vi "Live_Plot.vi"() -> ()   [LabVIEW 2013]
uses:
  Private/Controls/Graph.ctl
  Private/Controls/Constraints.ctl
  Private/Controls/Waveforms.ctl
  <vilib>/Utility/miscctls.llb/LVPointTypeDef.ctl
  <userlib>/_OpenG.lib/comparison/comparison.llb/Variant Changed__ogtk.vi
  <userlib>/_OpenG.lib/array/array.llb/Empty 1D Array (Variant)__ogtk.vi
panel:
  out "Cursor grabbed?":bool
  out "Month":dbl
  out "Updating...":bool
  out "Density (g/cc)":dbl=7.874000072479248 min=0.0 max=25.0
  in  "Tab Control":T1(tab)
  out "Number of Matching Events:":i64
  out "Percent of triggers that fit constraints:":dbl format="%#_4g%"
  out "Total Number of triggers:":i64
  in  "Enable\nTimestamp":bool
  out "Constrained Distribution":T2
  in  "Save Image":bool
  in  "Constraints":T3={"Upper Timestamp Range"=timestamp(0 s since 1904-01-01), "Lower Timestamp Range"=timestamp(0 s since 1904-01-01), "Experiment Group:"="", "Experiment Name:"=[], "Upper Velocity Limit (km/s)"=0.0, "Lower Velocity Limit (km/s)"=0.0, "Upper Mass Limit (kg)"=0.0, "Lower Mass Limit (kg)"=0.0, "name array"=[], "Estimate Quality"={0.0, 5.0}} {"Estimate Quality" scale=0.0..5.0; "Lower Mass Limit (kg)" min=0.0 step=1e-20; "Upper Mass Limit (kg)" min=0.0 step=1e-20}
  in  "Velocity":dbl=1.0 min=0.1 max=100.0
  in  "Mass":dbl=2.638602750087072e-13 min=1e-20 max=1e-10
  in  "Radius (µm)":dbl=2.0 min=0.00671912 max=14.4759
  in  "Reset Visible Time":bool caption="Save Metadata"
  in  "Time Visible":dbl=5000.0 min=0.0 max=5000.0 step=100.0
  out "Selected Waveforms":u64[](array[numeric])
  out "Waveforms":T4[](array[typedef])
  out "Max Time":dbl=5000.0
  in  "If this was the big acc...":bool
  out "Max Query Time":dbl
  in  "Pelletron Voltage (MV):":dbl=2.0
  out "Experiment Start":timestamp
  out "Test":bool caption="Test Database in use:"
  out "Test 2":bool caption="Production Database in use:"
  in  "error in (no error)":errorcluster
  out "error out":errorcluster
  in  "Vnoise Estimate:":dbl=0.005
  in  "Sensitivity:":dbl=12100000000000.0
  in  "Update interval (s)":dbl=5.0 min=1.0 max=60.0 step=1.0 format="%#_4g"
  out "Query Time":dbl
  in  "Small?":bool
  in  "Exit":bool
  # "Live Plot of Current Experiment"
  # "Cursor"
  # "Plot Settings:"
  # "ODBC Connection Status:"
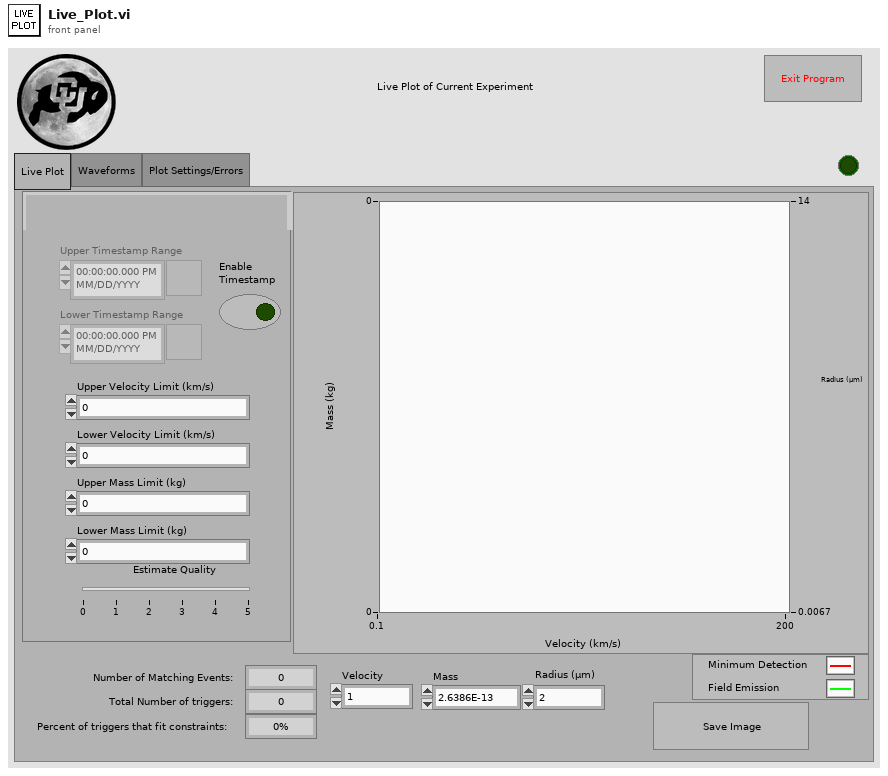
[diagram p1: front panel]
types:
  T1 = enum32{"Live Plot", "Waveforms", "Plot Settings/Errors"}
  T2 = typedef "Graph.ctl" = cluster{cluster{"Vnoise":dbl, "Vnoise":dbl}[]}[]
  T3 = typedef "Constraints.ctl" = cluster{"Upper Timestamp Range":timestamp, "Lower Timestamp Range":timestamp, "Experiment Group:":string, "Experiment Name:":i32[], "Upper Velocity Limit (km/s)":dbl, "Lower Velocity Limit (km/s)":dbl, "Upper Mass Limit (kg)":dbl, "Lower Mass Limit (kg)":dbl, "name array":string[], "Estimate Quality":cluster{dbl, dbl}}
  T4 = typedef "Waveforms.ctl" = cluster{"id_dust_event":u64, "Time Stamp":timestamp, "Velocity":dbl, "Mass":dbl, "Charge":dbl, "Radius":dbl, "Waveform Graph":sgl[][], "Quality":i32}
  T5 = typedef "LVPointTypeDef.ctl" = cluster{"Horizontal":i16, "Vertical":i16}
  T6 = typedef "LVRectTypeDef.ctl" = cluster{"Left":i16, "Top":i16, "Right":i16, "Bottom":i16}
  T7 = enum8{"Enabled", "Disabled", "Disabled and Grayed Out"}
  T8 = typedef "NI_Database_API.lvlib/Conn ObjectReference.ctl" = refnum<k1>
  T9 = typedef "Query_Dust_Event.ctl" = cluster{"Dust Event ID":i64, "Integer Timestamp":i64, "Velocity":sgl, "Mass":sgl, "Charge":sgl, "Radius":sgl, "Passed_3rd_Detector":i8, "High Voltage":sgl, "+ High Voltage Supply":sgl, "- High Voltage Supply":sgl, "HV Control Difference":sgl, "Vacuum Pressure":sgl, "Radiation":sgl, "Column Current":sgl, "Lost Charge":sgl, "Chain Current":sgl, "Control High Voltage":sgl, "Current Group Name:":string, "Current Experiment Name:":string, "Current Experiment Description:":string, "Estimate Source":T10, "Estimate Quality":i8, "File Location":T11, "Dust Type":string, "Dust Density":sgl}
  T10 = typedef "Estimate_source.ctl" = i8
  T11 = typedef "File_location.ctl" = i8
  T12 = typedef "imagedata.ctl" = cluster{"image type":i32, "image depth":i32, "image":u8[], "mask":u8[], "colors":u32[], "Rectangle":cluster{"left":i16, "top":i16, "right":i16, "bottom":i16}}
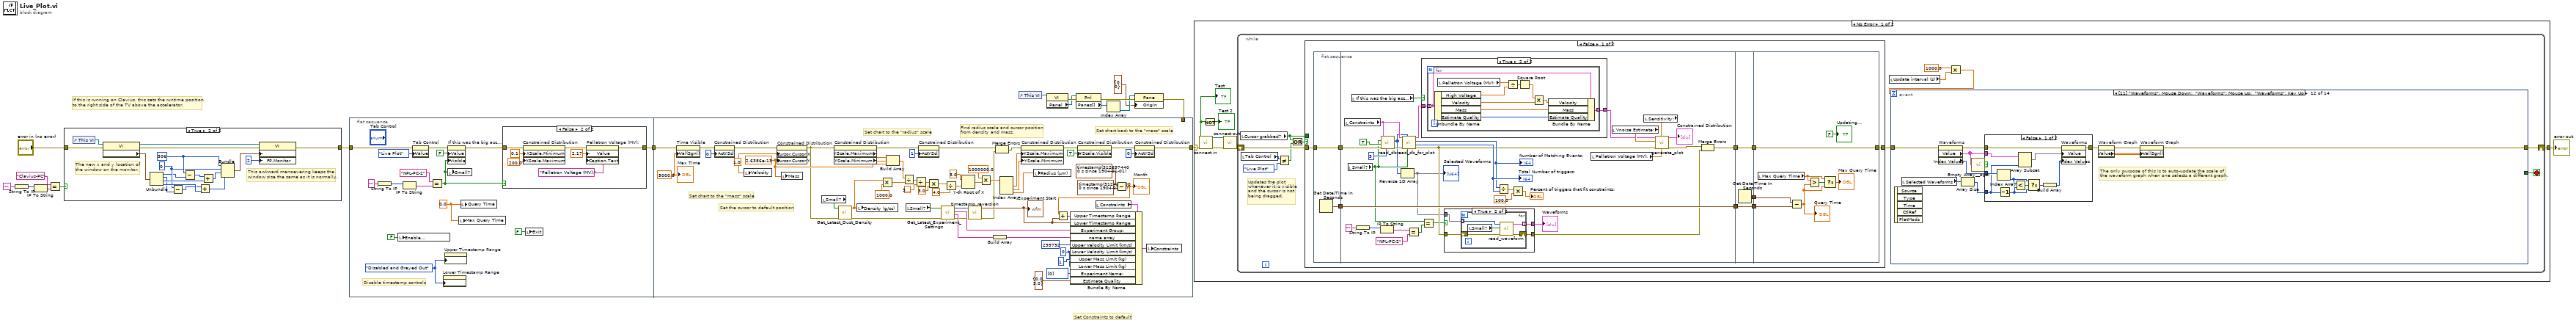
[diagram p0: block diagram]
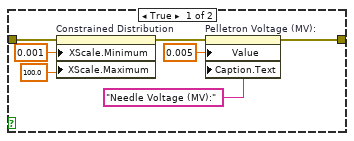
[diagram p3: hidden frame]
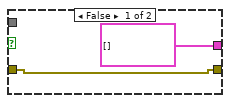
[diagram p4: hidden frame]
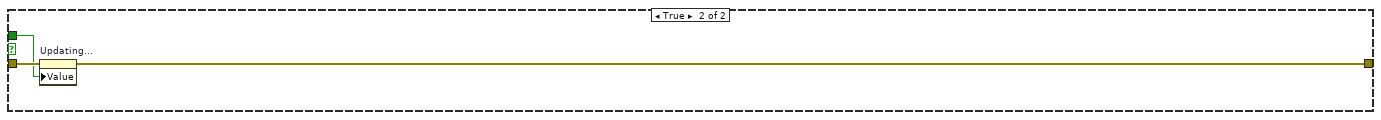
[diagram p6: hidden frame]
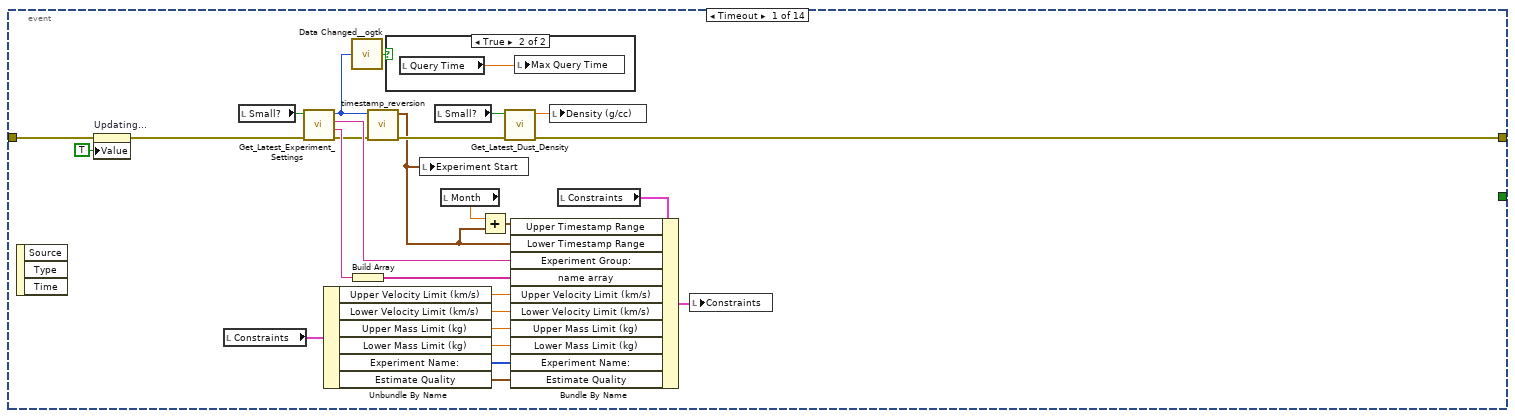
[diagram p7: hidden frame]
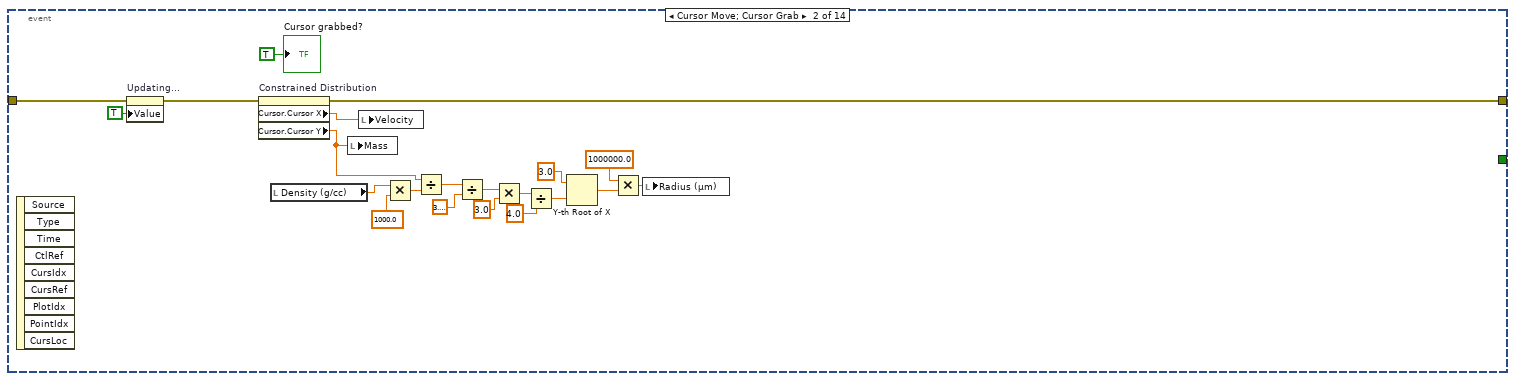
[diagram p9: hidden frame]
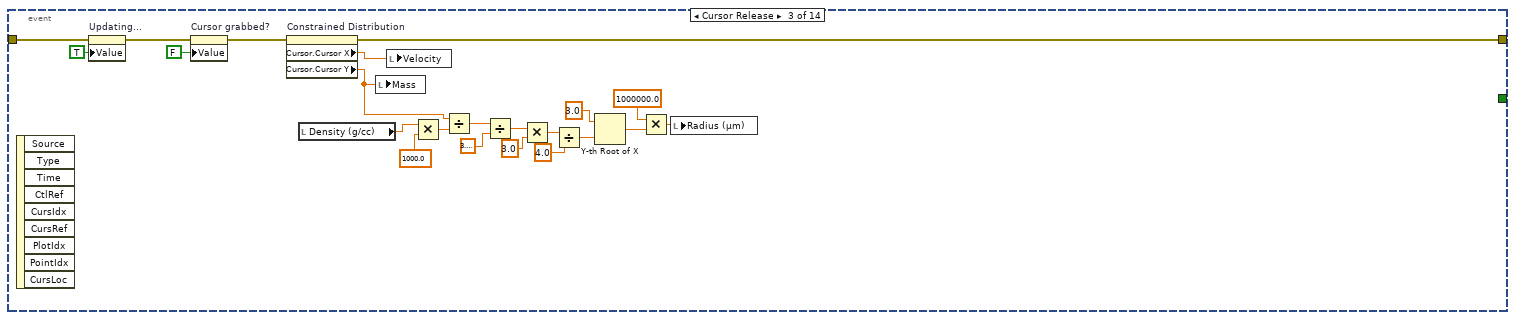
[diagram p10: hidden frame]
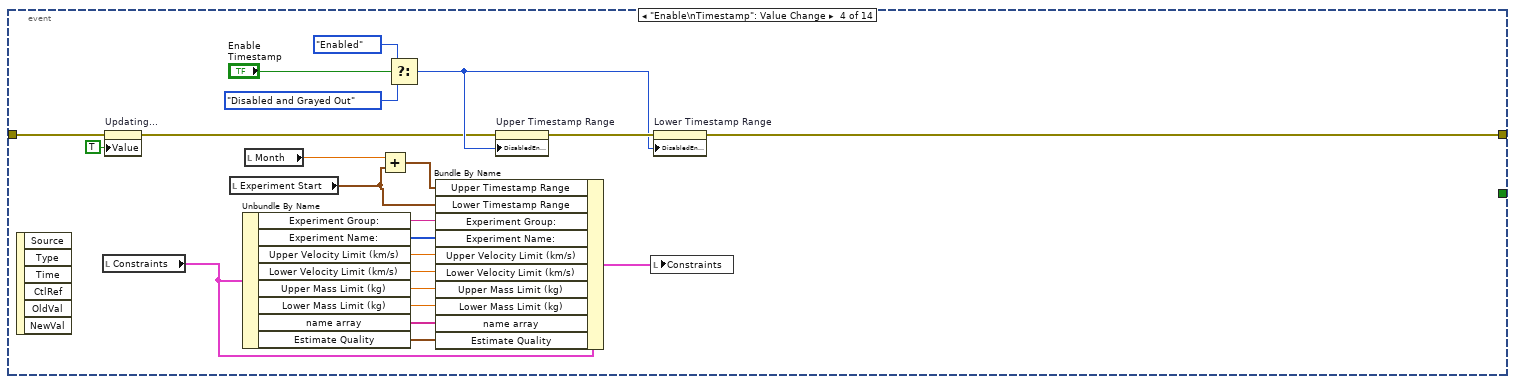
[diagram p11: hidden frame]
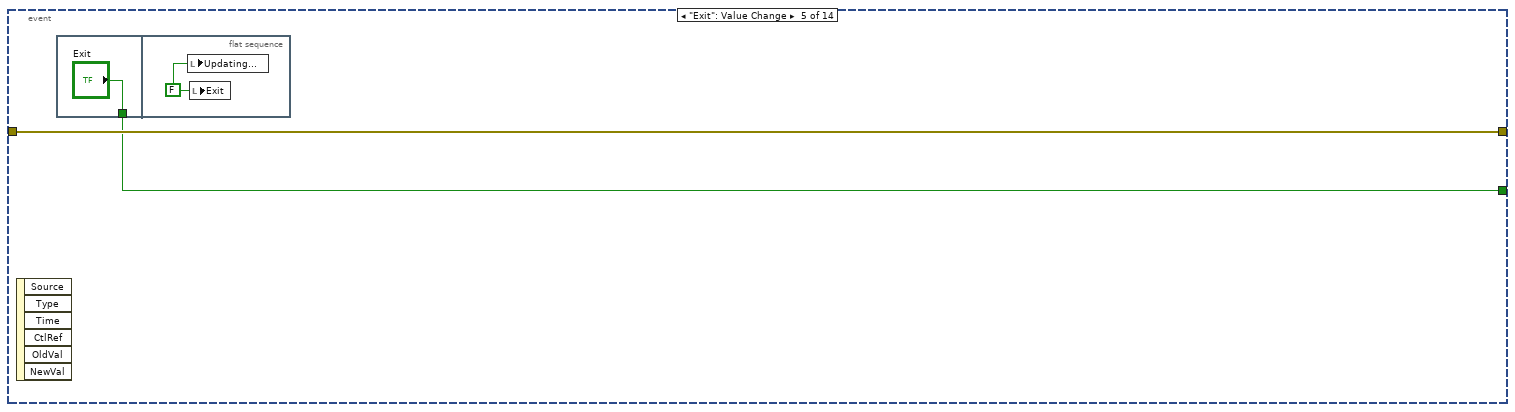
[diagram p12: hidden frame]
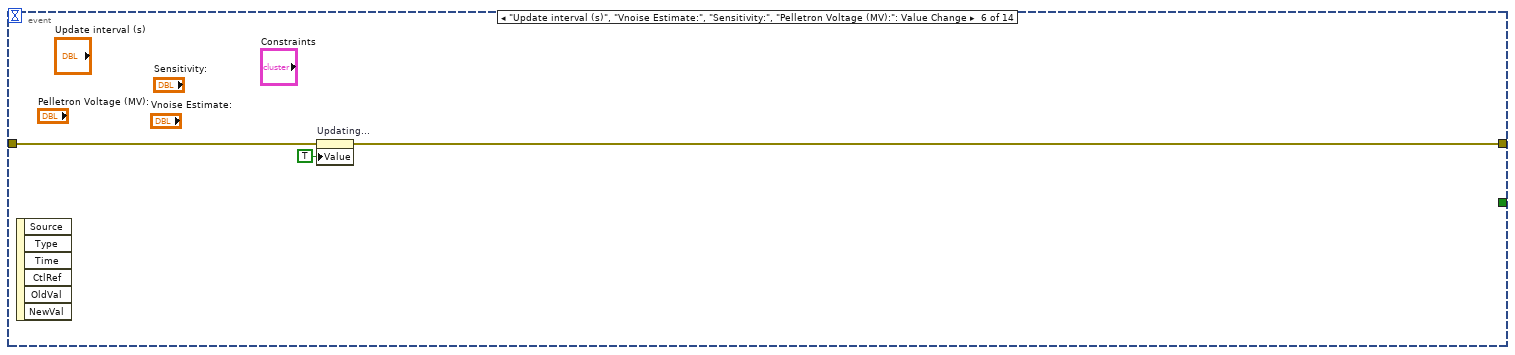
[diagram p13: hidden frame]
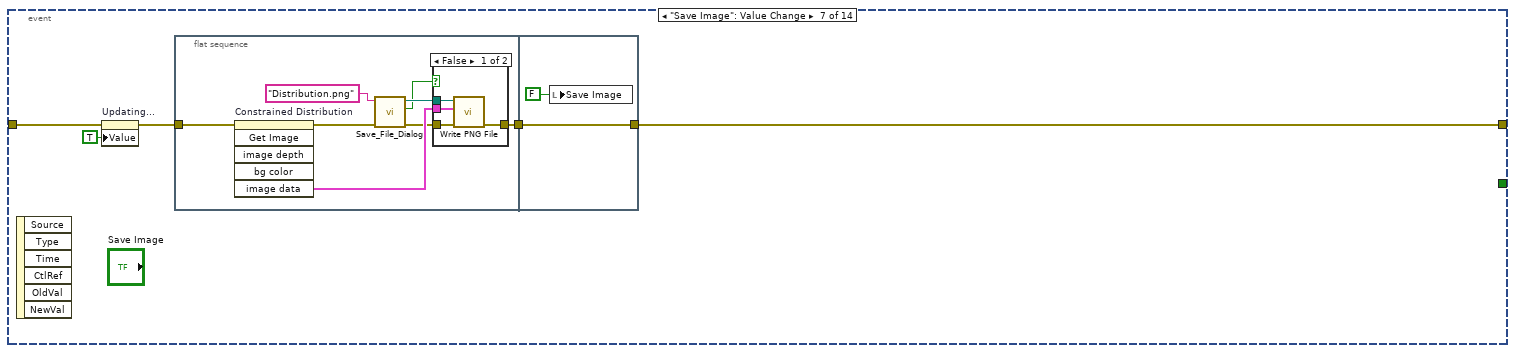
[diagram p14: hidden frame]
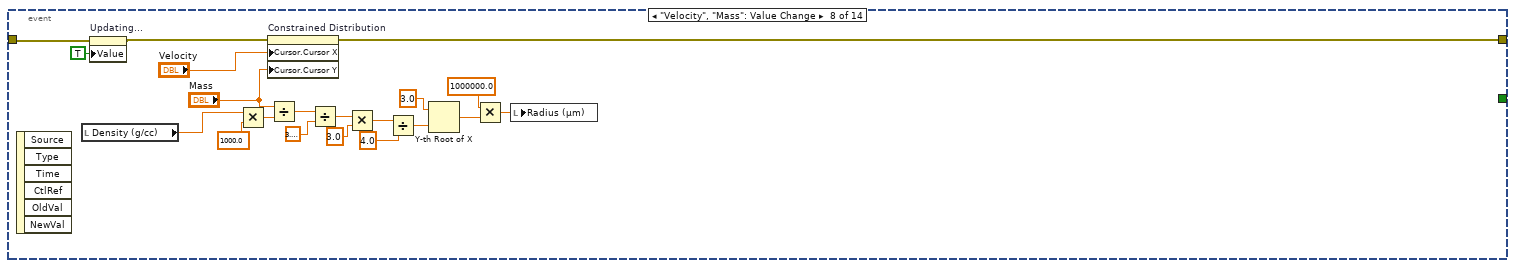
[diagram p16: hidden frame]
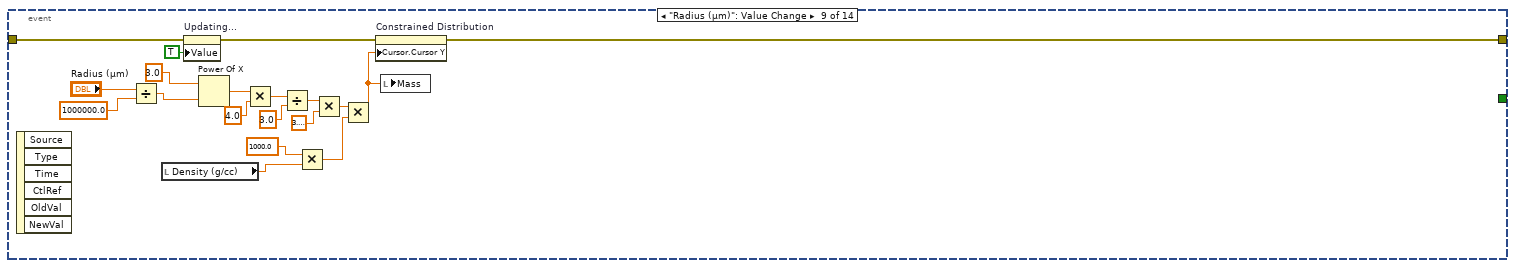
[diagram p17: hidden frame]
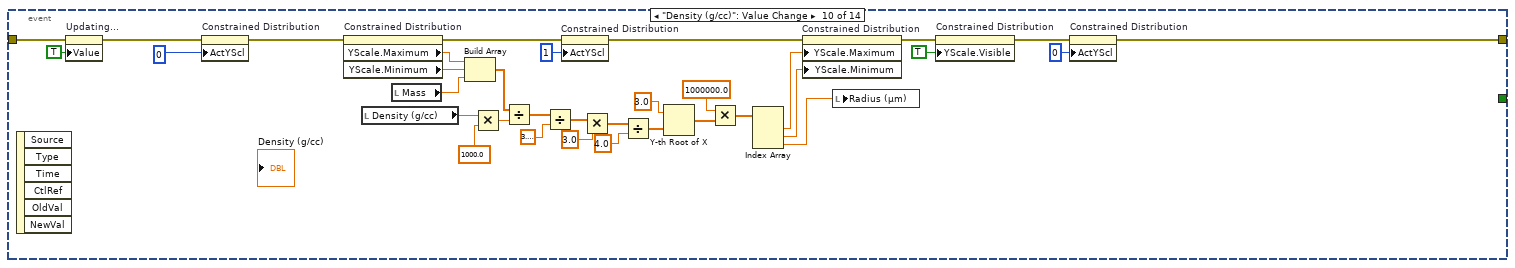
[diagram p18: hidden frame]
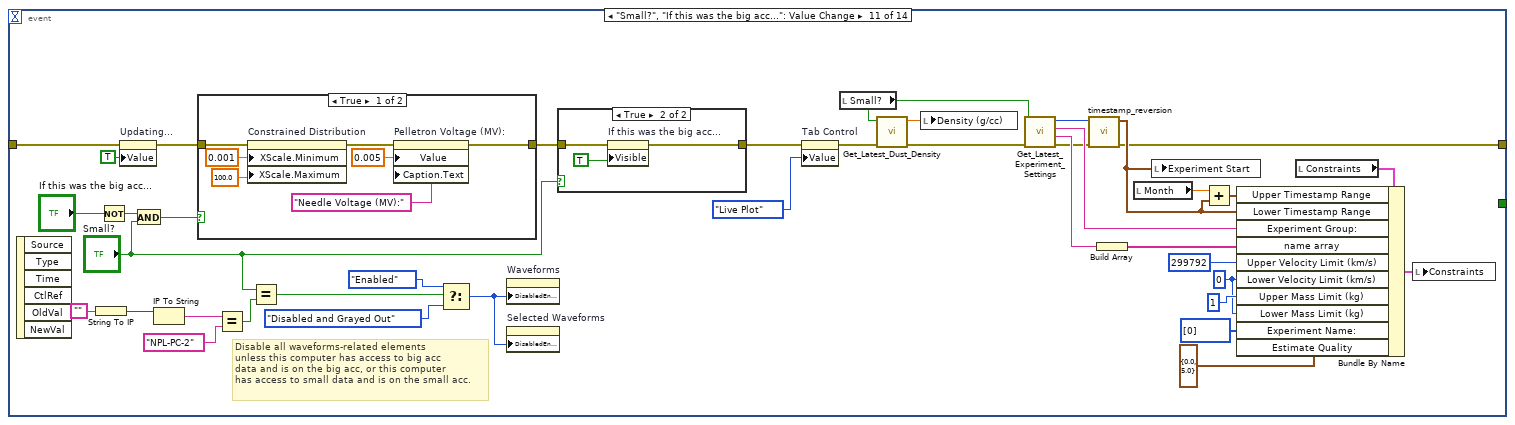
[diagram p19: hidden frame]
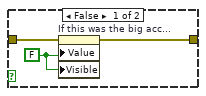
[diagram p20: hidden frame]
diagram:
  # "If this is running on Clavius, this sets the runtime position\nto the right side of the TV above the accelerator."
  # "Set Constraints to default"
  n1 = String To IP(1:"" ("name")) -> (0:w5:u32)
  n2 = IP To String(2:w5) -> (0:w3:string)  [unwired: 1 in]
  n3 = Equal?(x="Clavius-PC", y=w3) -> (x = y?=w7:bool)
  n4 = case shown="True" w7 {
    tunnel: "error in (no error)" -> [w19 w22]
    tunnel: [w19 w20] -> w1
    frame False {
    }
    frame True {
      w27 = i16 0 ("Top")
      w28 = i16 506 ("Left")
      # "This awkward manoevering keeps the\nwindow size the same as it is normally."
      # "The new x and y location of\nthe window on the monitor."
      n5 = control-ref of="This VI"() -> (w36:refnum<vi>)
      n6 = property class="VI"(reference=w36, error in=w22) -> (reference out=w32:refnum<vi>, error out=w21:errorcluster, "Front Panel.WinBounds"=w31:T6)
      n7 = Unbundle(w31) -> ("Left"=w26:i16, "Top"=w25:i16, "Right"=w30:i16, "Bottom"=w29:i16)
      n8 = Subtract(x=w27, y=w25) -> (x-y=w24:i16)
      n9 = Subtract(x=w28, y=w26) -> (x-y=w23:i16)
      n10 = Add(x=w24, y=w29) -> (x+y=w33:i16)
      n11 = Add(x=w23, y=w30) -> (x+y=w34:i16)
      n12 = Bundle("Left"=w28, "Top"=w27, w34, w33) -> (w37:cluster{"Left":i16, "Top":i16, i16, i16})  [unwired: 1 in]
      n13 = property class="VI"(reference=w32, error in=w21, "Front Panel.WinBounds"=w37, "FP.Monitor"=u16 2 ("Front Panel Window:Monitor")) -> (error out=w20:errorcluster)  [unwired: 1 out]
    }
  }
  n14 = flat-sequence {
    tunnel: [w48] -> w8
    tunnel: w1 -> [w40]
    tunnel: [w124] -> w10
    tunnel: w9 -> [_]
    tunnel: w8 -> [w69]
    frame #0 {
      w41 = 0.0 ("Query Time")
      w45 = T7."Disabled and Grayed Out" ("Disabled")
      # "Disable timestamp controls"
      n15 = String To IP(1:"" ("name")) -> (0:w51:u32)
      n16 = local write "Enable\nTimestamp"(FALSE ("Enable\nTimestamp")) -> ()
      n17 = IP To String(2:w51) -> (0:w49:string)  [unwired: 1 in]
      n18 = property on="Tab Control" class="TabCtl (strict)"(error in=w40, "Value"=T1."Live Plot" ("Tab Control")) -> (error out=w39:errorcluster)  [unwired: 1 in, 1 out]
      n19 = Equal?(x="NPL-PC-2", y=w49) -> (x = y?=w42:bool)
      n20 = property on="Lower Timestamp Range" class="AbsTime (strict)"("DisabledEnum"=w45) -> ()  [unwired: 2 in, 2 out]
      n21 = property on="Upper Timestamp Range" class="AbsTime (strict)"("DisabledEnum"=w45) -> ()  [unwired: 2 in, 2 out]
      n22 = property on="If this was the big acc..." class="Bool (strict)"(error in=w39, "Value"=FALSE ("If this was the big acc..."), "Visible"=w42) -> (error out=w44:errorcluster)  [unwired: 1 in, 1 out]
      n23 = local write "Small?"(w42) -> ()
      n24 = local write "Max Query Time"(w41) -> ()
      n25 = local write "Query Time"(w41) -> ()
      n26 = case shown="False" w42 {
        tunnel: [w57 w64] -> w48
        tunnel: w44 -> [w54 w61]
        frame True {
          n27 = property on="Constrained Distribution" class="XYGraph (strict)"(error in=w54, "XScale.Minimum"=0.001 ("X Scale.Range:Minimum"), "XScale.Maximum"=100.0 ("X Scale.Range:Maximum")) -> (error out=w53:errorcluster)  [unwired: 1 in, 1 out]
          n28 = property on="Pelletron Voltage (MV):" class="DigNum (strict)"(error in=w53, "Value"=0.005 ("Pelletron Voltage (MV):"), "Caption.Text"="Needle Voltage (MV):") -> (error out=w57:errorcluster)  [unwired: 1 in, 1 out]
        }
        frame False {
          n29 = property on="Constrained Distribution" class="XYGraph (strict)"(error in=w61, "XScale.Minimum"=0.1 ("X Scale.Range:Minimum"), "XScale.Maximum"=200.0 ("X Scale.Range:Maximum")) -> (error out=w60:errorcluster)  [unwired: 1 in, 1 out]
          n30 = property on="Pelletron Voltage (MV):" class="DigNum (strict)"(error in=w60, "Value"=2.17 ("Pelletron Voltage (MV):"), "Caption.Text"="Pelletron Voltage (MV):") -> (error out=w64:errorcluster)  [unwired: 1 in, 1 out]
        }
      }
      n31 = local write "Exit"(FALSE ("Exit")) -> ()
    }
    frame #1 {
      w67 = 5000.0 ("Max Time")
      w123 = 2.6386e-13 ("Mass")
      w107 = 1.0 ("Velocity")
      w116 = 0
      # "Set chart back to the \"mass\" scale"
      # "Set chart to the \"radius\" scale"
      # "Set chart to the \"mass\" scale"
      # "Find radius scale and cursor position\nfrom density and mass."
      # "Set the cursor to default position"
      n32 = property on="Time Visible" class="DigNum (strict)"(error in=w69, "Val(Sgnl)"=w67) -> (error out=w68:errorcluster)  [unwired: 1 in, 1 out]
      n33 = property on="Constrained Distribution" class="XYGraph (strict)"(error in=w68, "ActYScl"=0 ("Active Y Scale")) -> (error out=w75:errorcluster)  [unwired: 1 in, 1 out]
      n34 = local write "Velocity"(w107) -> ()
      n35 = property on="Constrained Distribution" class="XYGraph (strict)"(error in=w75, "Cursor.Cursor X"=w107, "Cursor.Cursor Y"=w123) -> (error out=w77:errorcluster)  [unwired: 1 in, 1 out]
      n36 = local write "Mass"(w123) -> ()
      n37 = local read "Small?"() -> (w74:bool)
      n38 = property on="Constrained Distribution" class="XYGraph (strict)"(error in=w77) -> (error out=w94:errorcluster, "YScale.Maximum"=w93:dbl, "YScale.Minimum"=w92:dbl)  [unwired: 1 in, 1 out]
      n39 = call "Get_Latest_Dust_Density.vi"("error in (no error)"=w77, "Small?"=w74) -> ("error out"=w79:errorcluster, "Density"=w78:dbl)  [unwired: 8 in]
      n40 = local write "Density (g/cc)"(w78) -> ()
      n41 = Multiply(x=w78, y=1000.0) -> (x*y=w98:dbl)
      n42 = Build Array(w93, w92, w123) -> (w91:dbl[])
      n43 = Divide(x=w91, y=w98) -> (x/y=w106:dbl[])
      n44 = local read "Small?"() -> (w73:bool)
      n45 = Divide(x=w106, y=3.141592653589793) -> (x/y=w104:dbl[])
      n46 = property on="Constrained Distribution" class="XYGraph (strict)"(error in=w94, "ActYScl"=1 ("Active Y Scale")) -> (error out=w90:errorcluster)  [unwired: 1 in, 1 out]
      n47 = Multiply(x=w104, y=3.0) -> (x*y=w102:dbl[])
      n48 = call "Get_Latest_Experiment_Settings.vi"("error in (no error)"=w79, "Small?"=w73) -> ("error out"=w80:errorcluster, "Experiment"=w110:string, "Group"=w109:string, "Integer Timestamp"=w108:i64)  [unwired: 5 in, 1 out]
      n49 = Divide(x=w102, y=4.0) -> (x/y=w100:dbl[])
      n50 = Y-th Root of X(1:w100, 2:3.0 ("y")) -> (0:w96:dbl[])
      n51 = call "timestamp_reversion.vi"("error in (no error)"=w80, "Integer Timestamp"=w108) -> ("error out"=w71:errorcluster, "time stamp"=w111:timestamp)  [unwired: 7 in]
      "Experiment Start" <- w111
      n52 = Multiply(x=1000000.0, y=w96) -> (x*y=w88:dbl[])
      n53 = Build Array(w110) -> (w70:string[])
      n54 = Merge Errors(w90, w71) -> (w72:errorcluster)
      n55 = Index Array(array=w88) -> (element #1=w86:dbl, element #2=w85:dbl, element #3=w84:dbl)  [unwired: 3 in]
      n56 = property on="Constrained Distribution" class="XYGraph (strict)"(error in=w72, "YScale.Maximum"=w86, "YScale.Minimum"=w85) -> (error out=w87:errorcluster)  [unwired: 1 in, 1 out]
      n57 = local write "Radius (µm)"(w84) -> ()
      n58 = property on="Constrained Distribution" class="XYGraph (strict)"(error in=w87, "YScale.Visible"=TRUE ("Y Scale.Visible")) -> (error out=w82:errorcluster)  [unwired: 1 in, 1 out]
      n59 = local read "Constraints"() -> (w122:T3)
      n60 = Subtract(x=timestamp(3126974400 s since 1904-01-01) ("current time"), y=timestamp(3124296000 s since 1904-01-01) ("current time")) -> (x-y=w119:dbl)
      "Month" <- w119
      n61 = Add(x=w119, y=w111) -> (x+y=w120:timestamp)
      n62 = Bundle By Name(cluster=w122, "Upper Timestamp Range"=w120, "Lower Timestamp Range"=w111, "Experiment Group:"=w109, "name array"=w70, "Upper Velocity Limit (km/s)"=299792, "Lower Velocity Limit (km/s)"=w116, "Upper Mass Limit (kg)"=1, "Lower Mass Limit (kg)"=w116, "Experiment Name:"=i32[] [0], "Estimate Quality"=cluster{dbl, dbl} {0.0, 5.0}) -> (w121:T3)
      n63 = property on="Constrained Distribution" class="XYGraph (strict)"(error in=w82, "ActYScl"=0 ("Active Y Scale")) -> (error out=w124:errorcluster)  [unwired: 1 in, 1 out]
      n64 = local write "Constraints"(w121) -> ()
      "Max Time" <- w67
    }
  }
  n65 = control-ref of="This VI"() -> (w17:refnum<vi>)
  n66 = property class="VI"(reference=w17) -> (error out=w16:errorcluster, "Panel"=w15:refnum<vi>)  [unwired: 1 in, 1 out]
  n67 = property class="Pnl"(reference=w15, error in=w16) -> (error out=w14:errorcluster, "Panes[]"=w13:refnum<vi>[])  [unwired: 1 out]
  n68 = Index Array(array=w13) -> (element=w12:refnum<vi>)  [unwired: 1 in]
  n69 = property class="Pane"(reference=w12, error in=w14, "Origin"=T5 {"Horizontal"=0, "Vertical"=0}) -> (error out=w9:errorcluster)  [unwired: 1 out]
  n70 = case shown="No Error" w10 {
    selector: w10 -> [w129 w520]
    tunnel: [w127 w520] -> w18
    frame No Error {
      n71 = call "connect in.vi"("error in (no error)"=w129) -> ("error out"=w130:errorcluster, "Database Connection"=w131:T8, "Test Server"=w128:bool)  [unwired: 6 in]
      "Test" <- w128
      n72 = Not(x=w128) -> (.not. x?=→"Test 2":bool)
      n73 = call "connect out.vi"("error in (no error)"=w130, "connection reference"=w131) -> ("error out"=w126:errorcluster)  [unwired: 9 in]
      n74 = while {
        shift-right: [w140] -> w127
        shift-left: w126 -> [w138]
        stop <- w141 stop-if-true
        # "Updates the plot\nwhenever it is visible\nand the cursor is not\nbeing dragged."
        n75 = local read "Cursor grabbed?"() -> (w132:bool)
        n76 = local read "Tab Control"() -> (w136:T1)
        n77 = Not Equal?(x=w136, y=T1."Live Plot") -> (x != y?=w134:bool)
        n78 = Or(x=w132, y=w134) -> (x .or. y?=w135:bool)
        n79 = case shown="False" w135 {
          tunnel: [w145 w222] -> w139
          tunnel: w138 -> [w144 w224]
          tunnel: w132 -> [_ w223]
          frame False {
            n80 = flat-sequence {
              tunnel: w144 -> [w154]
              tunnel: [w154] -> w152
              tunnel: [w153] -> w151
              tunnel: w152 -> [w173]
              tunnel: [w158] -> w150
              tunnel: [w178] -> w149
              tunnel: w151 -> [w178]
              tunnel: w150 -> [w213]
              tunnel: [w213] -> w148
              tunnel: w149 -> [w212]
              tunnel: [w212] -> w147
              tunnel: [w211] -> w146
              tunnel: [w221] -> w145
              tunnel: w148 -> [w221]
              tunnel: w147 -> [w220]
              tunnel: w146 -> [w215]
              frame #0 {
                n81 = Get Date/Time In Seconds() -> (seconds since 1Jan1904=w153:timestamp)
              }
              frame #1 {
                n82 = local read "Constraints"() -> (w171:T3)
                n83 = local read "Small?"() -> (w162:bool)
                n84 = local read "If this was the big acc..."() -> (w174:bool)
                n85 = String To IP(1:"" ("name")) -> (0:w165:u32)
                n86 = IP To String(2:w165) -> (0:w163:string)  [unwired: 1 in]
                n87 = call "read_db.vi"("No. of Events"=u64 5 ("Limit no. of events"), "error in (no error)"=w173, "Limited?"=TRUE, "Small?"=w162, "Constraints"=w171) -> ("error out"=w172:errorcluster, "Dust Event ID Array"=w156:i64[])  [unwired: 2 in, 3 out]
                n88 = Reverse 1D Array(array=w156) -> (reversed array=w155:i64[])
                "Selected Waveforms" <- w155
                n89 = call "read_db_for_plot.vi"("Small?"=w162, "Selected Dust Events"=w156, "error in (no error)"=w172, "Constraints"=w171) -> ("error out"=w168:errorcluster, "Total Number of triggers"=w179:u64, "Number of Matching Events"=w177:u64, "Dust Array"=w176:T9[])  [unwired: 3 in, 1 out]
                "Total Number of triggers:" <- w179
                "Number of Matching Events:" <- w177
                n90 = Equal?(x=w163, y="NPL-PC-2" ("x")) -> (x = y?=w167:bool)
                n91 = case shown="True" w174 {
                  tunnel: w176 -> [w198 w200]
                  tunnel: [w198 w199] -> w175
                  frame False {
                  }
                  frame True {
                    n92 = for {
                      tunnel: w200 -> [w210] mode=indexing
                      tunnel: [w209] -> w199 mode=indexing
                      n93 = Unbundle By Name(w210) -> ("High Voltage"=w205:sgl, "Velocity"=w204:sgl, "Mass"=w207:sgl, "Estimate Quality"=w208:i8)
                      n94 = local read "Pelletron Voltage (MV):"() -> (w206:dbl)
                      n95 = Divide(x=w206, y=w205) -> (x/y=w202:dbl)
                      n96 = Square Root(x=w202) -> (sqrt(x)=w201:dbl)
                      n97 = Multiply(x=w201, y=w204) -> (x*y=w203:dbl)
                      n98 = Bundle By Name(cluster=w210, "Velocity"=w203, "Mass"=w207, "Estimate Quality"=w208) -> (w209:T9)
                    }
                  }
                }
                n99 = Equal?(x=w162, y=w167) -> (x = y?=w161:bool)
                n100 = case shown="True" w161 {
                  tunnel: w168 -> [w187 w192]
                  tunnel: [T4[] [] ("Waveforms") w191] -> w160
                  tunnel: [w187 w190] -> w157
                  tunnel: w155 -> [_ w189]
                  frame False {
                  }
                  frame True {
                    n101 = for {
                      tunnel: [w195] -> w191 mode=indexing
                      shift-right: [w194] -> w190
                      shift-left: w192 -> [w196]
                      tunnel: w189 -> [w193] mode=indexing
                      n102 = local read "Small?"() -> (w197:bool)
                      n103 = call "read_waveform.vi"("error in (no error)"=w196, "Small?"=w197, "Dust Event ID"=w193) -> ("error out"=w194:errorcluster, "Waveform"=w195:T4)  [unwired: 7 in]
                    }
                  }
                }
                "Waveforms" <- w160
                n104 = Divide(x=w177, y=w179) -> (x/y=w182:dbl)
                n105 = Multiply(x=w182, y=100.0) -> (x*y=→"Percent of triggers that fit constraints:":dbl)
                n106 = local read "Pelletron Voltage (MV):"() -> (w183:dbl)
                n107 = local read "Vnoise Estimate:"() -> (w184:dbl)
                n108 = local read "Sensitivity:"() -> (w185:dbl)
                n109 = call "generate_plot.vi"("High Voltage"=w183, "Sens"=w185, "error in"=w168, "Vnoise"=w184, "Dust Array"=w175) -> ("error out"=w159:errorcluster, "Dust Distribution"=→"Constrained Distribution":T2)  [unwired: 5 in]
                n110 = Merge Errors(w159, w157) -> (w158:errorcluster)
              }
              frame #2 {
                n111 = Get Date/Time In Seconds() -> (seconds since 1Jan1904=w211:timestamp)
              }
              frame #3 {
                n112 = local read "Max Query Time"() -> (w218:dbl)
                n113 = Subtract(x=w215, y=w220) -> (x-y=w217:dbl)
                "Query Time" <- w217
                n114 = Greater?(x=w218, y=w217) -> (0:w219:bool)
                n115 = Select(t=w218, s=w219, f=w217) -> (s? t:f=→"Max Query Time":dbl)
                "Updating..." <- FALSE ("Updating...")
              }
            }
          }
          frame True {
            n116 = property on="Updating..." class="Bool (strict)"(error in=w224, "Value"=w223) -> (error out=w222:errorcluster)  [unwired: 1 in, 1 out]
          }
        }
        n117 = local read "Update interval (s)"() -> (w137:dbl)
        n118 = Multiply(x=1000.0, y=w137) -> (x*y=w142:dbl)
        n119 = event shown="[11] \"Waveforms\": Mouse Down;  \"Waveforms\": Mouse Up;  \"Waveforms\": Key Up" {
          selector: _ -> [_ _ _ _ _ _ _ _ _ _ _ _ _ _]
          dyn-events: _ -> [_ _ _ _ _ _ _ _ _ _ _ _ _ _]
          timeout: w142 -> [_ _ _ _ _ _ _ _ _ _ _ _ _ _]
          tunnel: w139 -> [w226 w252 w274 w296 w318 w323 w324 w344 w364 w385 w430 w481 w502 w507]
          tunnel: [w250 w256 w276 w303 w318 w322 w328 w363 w382 w389 w438 w484 w500 w503] -> w140
          tunnel: [_ _ _ _ w317 _ _ _ _ _ _ _ _ _] -> w141
          event Timeout {
            n120 = event-data() -> ()  [unwired: 1 in, 3 out]
            n121 = property on="Updating..." class="Bool (strict)"(error in=w226, "Value"=TRUE ("Updating...")) -> (error out=w227:errorcluster)  [unwired: 1 in, 1 out]
            n122 = local read "Constraints"() -> (w240:T3)
            n123 = local read "Small?"() -> (w231:bool)
            n124 = call "Get_Latest_Experiment_Settings.vi"("error in (no error)"=w227, "Small?"=w231) -> ("error out"=w244:errorcluster, "Experiment"=w246:string, "Group"=w245:string, "Integer Timestamp"=w233:i64)  [unwired: 5 in, 1 out]
            n125 = Unbundle By Name(w240) -> ("Upper Velocity Limit (km/s)"=w239:dbl, "Lower Velocity Limit (km/s)"=w238:dbl, "Upper Mass Limit (kg)"=w237:dbl, "Lower Mass Limit (kg)"=w236:dbl, "Experiment Name:"=w235:i32[], "Estimate Quality"=w234:cluster{dbl, dbl})
            n126 = call-poly <userlib>:"Data Changed__ogtk.vi"("Variant"=w233) -> ("Changed"=w232:bool)
            n127 = Build Array(w246) -> (w225:string[])
            n128 = call "timestamp_reversion.vi"("error in (no error)"=w244, "Integer Timestamp"=w233) -> ("error out"=w242:errorcluster, "time stamp"=w229:timestamp)  [unwired: 7 in]
            n129 = case shown="True" w232 {
              frame False {
              }
              frame True {
                n130 = local read "Query Time"() -> (w251:dbl)
                n131 = local write "Max Query Time"(w251) -> ()
              }
            }
            n132 = local write "Experiment Start"(w229) -> ()
            n133 = local read "Small?"() -> (w230:bool)
            n134 = local read "Month"() -> (w243:dbl)
            n135 = Add(x=w243, y=w229) -> (x+y=w247:timestamp)
            n136 = call "Get_Latest_Dust_Density.vi"("error in (no error)"=w242, "Small?"=w230) -> ("error out"=w250:errorcluster, "Density"=w241:dbl)  [unwired: 8 in]
            n137 = local write "Density (g/cc)"(w241) -> ()
            n138 = local read "Constraints"() -> (w249:T3)
            n139 = Bundle By Name(cluster=w249, "Upper Timestamp Range"=w247, "Lower Timestamp Range"=w229, "Experiment Group:"=w245, "name array"=w225, "Upper Velocity Limit (km/s)"=w239, "Lower Velocity Limit (km/s)"=w238, "Upper Mass Limit (kg)"=w237, "Lower Mass Limit (kg)"=w236, "Experiment Name:"=w235, "Estimate Quality"=w234) -> (w248:T3)
            n140 = local write "Constraints"(w248) -> ()
          }
          event Cursor Move; Cursor Grab {
            n141 = event-data() -> ()  [unwired: 1 in, 9 out]
            n142 = property on="Updating..." class="Bool (strict)"(error in=w252, "Value"=TRUE ("Updating...")) -> (error out=w253:errorcluster)  [unwired: 1 in, 1 out]
            n143 = property on="Constrained Distribution" class="XYGraph (strict)"(error in=w253) -> (error out=w256:errorcluster, "Cursor.Cursor X"=w272:dbl, "Cursor.Cursor Y"=w259:dbl)  [unwired: 1 in, 1 out]
            n144 = local read "Density (g/cc)"() -> (w258:dbl)
            n145 = local write "Mass"(w259) -> ()
            n146 = local write "Velocity"(w272) -> ()
            n147 = Multiply(x=w258, y=1000.0) -> (x*y=w263:dbl)
            n148 = Divide(x=w259, y=w263) -> (x/y=w271:dbl)
            n149 = Divide(x=w271, y=3.141592653589793) -> (x/y=w269:dbl)
            n150 = Multiply(x=w269, y=3.0) -> (x*y=w267:dbl)
            n151 = Divide(x=w267, y=4.0) -> (x/y=w265:dbl)
            n152 = Y-th Root of X(1:w265, 2:3.0 ("y")) -> (0:w261:dbl)
            n153 = Multiply(x=1000000.0, y=w261) -> (x*y=w257:dbl)
            n154 = local write "Radius (µm)"(w257) -> ()
            "Cursor grabbed?" <- TRUE ("Updating...")
          }
          event Cursor Release {
            n155 = event-data() -> ()  [unwired: 1 in, 9 out]
            n156 = property on="Updating..." class="Bool (strict)"(error in=w274, "Value"=TRUE ("Updating...")) -> (error out=w273:errorcluster)  [unwired: 1 in, 1 out]
            n157 = property on="Cursor grabbed?" class="Bool (strict)"(error in=w273, "Value"=FALSE ("Cursor grabbed?")) -> (error out=w277:errorcluster)  [unwired: 1 in, 1 out]
            n158 = property on="Constrained Distribution" class="XYGraph (strict)"(error in=w277) -> (error out=w276:errorcluster, "Cursor.Cursor X"=w293:dbl, "Cursor.Cursor Y"=w280:dbl)  [unwired: 1 in, 1 out]
            n159 = local read "Density (g/cc)"() -> (w279:dbl)
            n160 = local write "Mass"(w280) -> ()
            n161 = local write "Velocity"(w293) -> ()
            n162 = Multiply(x=w279, y=1000.0) -> (x*y=w284:dbl)
            n163 = Divide(x=w280, y=w284) -> (x/y=w292:dbl)
            n164 = Divide(x=w292, y=3.141592653589793) -> (x/y=w290:dbl)
            n165 = Multiply(x=w290, y=3.0) -> (x*y=w288:dbl)
            n166 = Divide(x=w288, y=4.0) -> (x/y=w286:dbl)
            n167 = Y-th Root of X(1:w286, 2:3.0 ("y")) -> (0:w282:dbl)
            n168 = Multiply(x=1000000.0, y=w282) -> (x*y=w278:dbl)
            n169 = local write "Radius (µm)"(w278) -> ()
          }
          event "Enable\nTimestamp": Value Change {
            n170 = event-data() -> ()  [unwired: 1 in, 6 out]
            n171 = local read "Constraints"() -> (w316:T3)
            n172 = property on="Updating..." class="Bool (strict)"(error in=w296, "Value"=TRUE ("Updating...")) -> (error out=w297:errorcluster)  [unwired: 1 in, 1 out]
            n173 = local read "Experiment Start"() -> (w298:timestamp)
            n174 = Unbundle By Name(w316) -> ("Experiment Group:"=w307:string, "Experiment Name:"=w308:i32[], "Upper Velocity Limit (km/s)"=w309:dbl, "Lower Velocity Limit (km/s)"=w310:dbl, "Upper Mass Limit (kg)"=w311:dbl, "Lower Mass Limit (kg)"=w312:dbl, "name array"=w313:string[], "Estimate Quality"=w314:cluster{dbl, dbl})
            n175 = local read "Month"() -> (w305:dbl)
            n176 = Add(x=w305, y=w298) -> (x+y=w306:timestamp)
            n177 = Select(t=T7."Enabled" ("Disabled"), s="Enable\nTimestamp", f=T7."Disabled and Grayed Out" ("Disabled")) -> (s? t:f=w299:T7)
            n178 = Bundle By Name(cluster=w316, "Upper Timestamp Range"=w306, "Lower Timestamp Range"=w298, "Experiment Group:"=w307, "Experiment Name:"=w308, "Upper Velocity Limit (km/s)"=w309, "Lower Velocity Limit (km/s)"=w310, "Upper Mass Limit (kg)"=w311, "Lower Mass Limit (kg)"=w312, "name array"=w313, "Estimate Quality"=w314) -> (w315:T3)
            n179 = property on="Upper Timestamp Range" class="AbsTime (strict)"(error in=w297, "DisabledEnum"=w299) -> (error out=w304:errorcluster)  [unwired: 1 in, 1 out]
            n180 = local write "Constraints"(w315) -> ()
            n181 = property on="Lower Timestamp Range" class="AbsTime (strict)"(error in=w304, "DisabledEnum"=w299) -> (error out=w303:errorcluster)  [unwired: 1 in, 1 out]
          }
          event "Exit": Value Change {
            n182 = event-data() -> ()  [unwired: 1 in, 6 out]
            n183 = flat-sequence {
              tunnel: ["Exit"] -> w317
              frame #0 {
              }
              frame #1 {
                w320 = FALSE ("Exit")
                n184 = local write "Updating..."(w320) -> ()
                n185 = local write "Exit"(w320) -> ()
              }
            }
          }
          event "Update interval (s)", "Vnoise Estimate:", "Sensitivity:", "Pelletron Voltage (MV):": Value Change {
            n186 = event-data() -> ()  [unwired: 1 in, 6 out]
            n187 = property on="Updating..." class="Bool (strict)"(error in=w323, "Value"=TRUE ("Updating...")) -> (error out=w322:errorcluster)  [unwired: 1 in, 1 out]
          }
          event "Save Image": Value Change {
            n188 = event-data() -> ()  [unwired: 1 in, 6 out]
            n189 = property on="Updating..." class="Bool (strict)"(error in=w324, "Value"=TRUE ("Updating...")) -> (error out=w325:errorcluster)  [unwired: 1 in, 1 out]
            n190 = flat-sequence {
              tunnel: [w335] -> w327
              tunnel: w325 -> [w334]
              tunnel: [w343] -> w328
              tunnel: w327 -> [w343]
              frame #0 {
                n191 = invoke on="Constrained Distribution" class="XYGraph (strict)" method="Get Image"(error in=w334) -> (error out=w333:errorcluster, "image data"=w336:T12)  [unwired: 5 in, 4 out]
                n192 = call "Save_File_Dialog.vi"("error in (no error)"=w333, "Filename"="Distribution.png") -> ("error out"=w331:errorcluster, "Cancelled"=w329:bool, "Path"=w330:path)  [unwired: 7 in]
                n193 = case shown="False" w329 {
                  tunnel: w336 -> [w340 _]
                  tunnel: [w339 w341] -> w335
                  tunnel: w330 -> [w338 _]
                  tunnel: w331 -> [w337 w341]
                  frame False {
                    n194 = call <vilib>:"Write PNG File.vi"("error in (no error)"=w337, "image data"=w340, "path to PNG file"=w338) -> ("error out"=w339:errorcluster)  [unwired: 7 in, 1 out]
                  }
                  frame True {
                  }
                }
              }
              frame #1 {
                n195 = local write "Save Image"(FALSE ("Save Image")) -> ()
              }
            }
          }
          event "Velocity", "Mass": Value Change {
            n196 = event-data() -> ()  [unwired: 1 in, 6 out]
            n197 = local read "Density (g/cc)"() -> (w361:dbl)
            n198 = property on="Updating..." class="Bool (strict)"(error in=w344, "Value"=TRUE ("Updating...")) -> (error out=w345:errorcluster)  [unwired: 1 in, 1 out]
            n199 = Multiply(x=w361, y=1000.0) -> (x*y=w352:dbl)
            n200 = property on="Constrained Distribution" class="XYGraph (strict)"(error in=w345, "Cursor.Cursor X"="Velocity", "Cursor.Cursor Y"="Mass") -> (error out=w363:errorcluster)  [unwired: 1 in, 1 out]
            n201 = Divide(x="Mass", y=w352) -> (x/y=w360:dbl)
            n202 = Divide(x=w360, y=3.141592653589793) -> (x/y=w358:dbl)
            n203 = Multiply(x=w358, y=3.0) -> (x*y=w356:dbl)
            n204 = Divide(x=w356, y=4.0) -> (x/y=w354:dbl)
            n205 = Y-th Root of X(1:w354, 2:3.0 ("y")) -> (0:w349:dbl)
            n206 = Multiply(x=1000000.0, y=w349) -> (x*y=w348:dbl)
            n207 = local write "Radius (µm)"(w348) -> ()
          }
          event "Radius (µm)": Value Change {
            n208 = event-data() -> ()  [unwired: 1 in, 6 out]
            n209 = Divide(x="Radius (µm)", y=1000000.0) -> (x/y=w373:dbl)
            n210 = local read "Density (g/cc)"() -> (w367:dbl)
            n211 = property on="Updating..." class="Bool (strict)"(error in=w364, "Value"=TRUE ("Updating...")) -> (error out=w365:errorcluster)  [unwired: 1 in, 1 out]
            n212 = Power Of X(1:w373, 2:3.0 ("y")) -> (0:w372:dbl)
            n213 = Multiply(x=w372, y=4.0) -> (x*y=w379:dbl)
            n214 = Divide(x=w379, y=3.0) -> (x/y=w377:dbl)
            n215 = Multiply(x=1000.0, y=w367) -> (x*y=w370:dbl)
            n216 = Multiply(x=w377, y=3.141592653589793) -> (x*y=w371:dbl)
            n217 = Multiply(x=w371, y=w370) -> (x*y=w368:dbl)
            n218 = property on="Constrained Distribution" class="XYGraph (strict)"(error in=w365, "Cursor.Cursor Y"=w368) -> (error out=w382:errorcluster)  [unwired: 1 in, 1 out]
            n219 = local write "Mass"(w368) -> ()
          }
          event "Density (g/cc)": Value Change {
            n220 = event-data() -> ()  [unwired: 1 in, 6 out]
            n221 = property on="Updating..." class="Bool (strict)"(error in=w385, "Value"=TRUE ("Updating...")) -> (error out=w383:errorcluster)  [unwired: 1 in, 1 out]
            n222 = property on="Constrained Distribution" class="XYGraph (strict)"(error in=w383, "ActYScl"=0 ("Active Y Scale")) -> (error out=w401:errorcluster)  [unwired: 1 in, 1 out]
            n223 = property on="Constrained Distribution" class="XYGraph (strict)"(error in=w401) -> (error out=w403:errorcluster, "YScale.Maximum"=w404:dbl, "YScale.Minimum"=w405:dbl)  [unwired: 1 in, 1 out]
            n224 = local read "Density (g/cc)"() -> (w399:dbl)
            n225 = local read "Mass"() -> (w390:dbl)
            n226 = Build Array(w404, w405, w390) -> (w406:dbl[])
            n227 = Multiply(x=w399, y=1000.0) -> (x*y=w397:dbl)
            n228 = Divide(x=w406, y=w397) -> (x/y=w391:dbl[])
            n229 = Divide(x=w391, y=3.141592653589793) -> (x/y=w393:dbl[])
            n230 = property on="Constrained Distribution" class="XYGraph (strict)"(error in=w403, "ActYScl"=1 ("Active Y Scale")) -> (error out=w407:errorcluster)  [unwired: 1 in, 1 out]
            n231 = Multiply(x=w393, y=3.0) -> (x*y=w394:dbl[])
            n232 = Divide(x=w394, y=4.0) -> (x/y=w395:dbl[])
            n233 = Y-th Root of X(1:w395, 2:3.0 ("y")) -> (0:w398:dbl[])
            n234 = Multiply(x=1000000.0, y=w398) -> (x*y=w409:dbl[])
            n235 = Index Array(array=w409) -> (element #1=w411:dbl, element #2=w412:dbl, element #3=w413:dbl)  [unwired: 3 in]
            n236 = property on="Constrained Distribution" class="XYGraph (strict)"(error in=w407, "YScale.Maximum"=w411, "YScale.Minimum"=w412) -> (error out=w410:errorcluster)  [unwired: 1 in, 1 out]
            n237 = local write "Radius (µm)"(w413) -> ()
            n238 = property on="Constrained Distribution" class="XYGraph (strict)"(error in=w410, "YScale.Visible"=TRUE ("Y Scale.Visible")) -> (error out=w415:errorcluster)  [unwired: 1 in, 1 out]
            n239 = property on="Constrained Distribution" class="XYGraph (strict)"(error in=w415, "ActYScl"=0 ("Active Y Scale")) -> (error out=w389:errorcluster)  [unwired: 1 in, 1 out]
          }
          event "Small?", "If this was the big acc...": Value Change {
            w448 = 0
            # "Disable all waveforms-related elements\nunless this computer has access to big acc\ndata and is on the big acc, or this computer\nhas access to small data and is on the small acc."
            n240 = event-data() -> ()  [unwired: 1 in, 6 out]
            n241 = String To IP(1:"" ("name")) -> (0:w425:u32)
            n242 = Not(x="If this was the big acc...") -> (.not. x?=w435:bool)
            n243 = property on="Updating..." class="Bool (strict)"(error in=w430, "Value"=TRUE ("Updating...")) -> (error out=w429:errorcluster)  [unwired: 1 in, 1 out]
            n244 = And(x=w435, y="Small?") -> (x .and. y?=w437:bool)
            n245 = IP To String(2:w425) -> (0:w427:string)  [unwired: 1 in]
            n246 = case shown="True" w437 {
              tunnel: [w466 w473] -> w434
              tunnel: w429 -> [w463 w470]
              frame True {
                n247 = property on="Constrained Distribution" class="XYGraph (strict)"(error in=w463, "XScale.Minimum"=0.001 ("X Scale.Range:Minimum"), "XScale.Maximum"=100.0 ("X Scale.Range:Maximum")) -> (error out=w462:errorcluster)  [unwired: 1 in, 1 out]
                n248 = property on="Pelletron Voltage (MV):" class="DigNum (strict)"(error in=w462, "Value"=0.005 ("Pelletron Voltage (MV):"), "Caption.Text"="Needle Voltage (MV):") -> (error out=w466:errorcluster)  [unwired: 1 in, 1 out]
              }
              frame False {
                n249 = property on="Constrained Distribution" class="XYGraph (strict)"(error in=w470, "XScale.Minimum"=0.1 ("X Scale.Range:Minimum"), "XScale.Maximum"=200.0 ("X Scale.Range:Maximum")) -> (error out=w469:errorcluster)  [unwired: 1 in, 1 out]
                n250 = property on="Pelletron Voltage (MV):" class="DigNum (strict)"(error in=w469, "Value"=2.17 ("Pelletron Voltage (MV):"), "Caption.Text"="Pelletron Voltage (MV):") -> (error out=w473:errorcluster)  [unwired: 1 in, 1 out]
              }
            }
            n251 = Equal?(x=w427, y="NPL-PC-2" ("x")) -> (x = y?=w422:bool)
            n252 = Equal?(x="Small?", y=w422) -> (x = y?=w419:bool)
            n253 = Select(t=T7."Enabled" ("Disabled"), s=w419, f=T7."Disabled and Grayed Out") -> (s? t:f=w418:T7)
            n254 = property on="Waveforms" class="Arr (strict)"("DisabledEnum"=w418) -> ()  [unwired: 2 in, 2 out]
            n255 = property on="Selected Waveforms" class="Arr (strict)"("DisabledEnum"=w418) -> ()  [unwired: 2 in, 2 out]
            n256 = case shown="True" "Small?" {
              tunnel: w434 -> [w458 w460]
              tunnel: [w457 w459] -> w433
              frame False {
                w456 = FALSE ("If this was the big acc...")
                n257 = property on="If this was the big acc..." class="Bool (strict)"(error in=w458, "Value"=w456, "Visible"=w456) -> (error out=w457:errorcluster)  [unwired: 1 in, 1 out]
              }
              frame True {
                n258 = property on="If this was the big acc..." class="Bool (strict)"(error in=w460, "Visible"=TRUE) -> (error out=w459:errorcluster)  [unwired: 1 in, 1 out]
              }
            }
            n259 = property on="Tab Control" class="TabCtl (strict)"(error in=w433, "Value"=T1."Live Plot" ("Tab Control")) -> (error out=w439:errorcluster)  [unwired: 1 in, 1 out]
            n260 = local read "Small?"() -> (w432:bool)
            n261 = call "Get_Latest_Dust_Density.vi"("error in (no error)"=w439, "Small?"=w432) -> ("error out"=w441:errorcluster, "Density"=w440:dbl)  [unwired: 8 in]
            n262 = local write "Density (g/cc)"(w440) -> ()
            n263 = call "Get_Latest_Experiment_Settings.vi"("error in (no error)"=w441, "Small?"=w432) -> ("error out"=w442:errorcluster, "Experiment"=w445:string, "Group"=w444:string, "Integer Timestamp"=w443:i64)  [unwired: 5 in, 1 out]
            n264 = call "timestamp_reversion.vi"("error in (no error)"=w442, "Integer Timestamp"=w443) -> ("error out"=w438:errorcluster, "time stamp"=w453:timestamp)  [unwired: 7 in]
            n265 = Build Array(w445) -> (w417:string[])
            n266 = local read "Month"() -> (w454:dbl)
            n267 = local write "Experiment Start"(w453) -> ()
            n268 = Add(x=w454, y=w453) -> (x+y=w450:timestamp)
            n269 = local read "Constraints"() -> (w452:T3)
            n270 = Bundle By Name(cluster=w452, "Upper Timestamp Range"=w450, "Lower Timestamp Range"=w453, "Experiment Group:"=w444, "name array"=w417, "Upper Velocity Limit (km/s)"=299792, "Lower Velocity Limit (km/s)"=w448, "Upper Mass Limit (kg)"=1, "Lower Mass Limit (kg)"=w448, "Experiment Name:"=i32[] [0], "Estimate Quality"=cluster{dbl, dbl} {0.0, 5.0}) -> (w451:T3)
            n271 = local write "Constraints"(w451) -> ()
          }
          event "Waveforms": Mouse Down; "Waveforms": Mouse Up; "Waveforms": Key Up {
            # "The only purpose of this is to auto-update the scale of\nthe waveform graph when one selects a different graph."
            n272 = event-data() -> ()  [unwired: 1 in, 5 out]
            n273 = local read "Selected Waveforms"() -> (w477:u64[])
            n274 = property on="Waveforms" class="Arr (strict)"(error in=w481) -> (error out=w480:errorcluster, "Value"=w478:T4[], "Index Values"=w482:u32[])  [unwired: 1 in, 1 out]
            n275 = Array Size(array=w477) -> (size(s)=w476:i32)
            n276 = call-poly <userlib>:"Empty Array__ogtk.vi"("Array"=w478) -> ("Empty Array?"=w483:bool)  [unwired: 8 in]
            n277 = case shown="False" w483 {
              tunnel: w482 -> [w493 _]
              tunnel: w480 -> [w492 w498]
              tunnel: [w491 w498] -> w479
              tunnel: w478 -> [w490 _]
              tunnel: w476 -> [w489 _]
              frame False {
                n278 = Index Array(array=w493) -> (element=w495:u32)  [unwired: 1 in]
                n279 = Decrement(x=w489) -> (x-1=w496:i32)
                n280 = Less?(x=w495, y=w496) -> (x < y?=w494:bool)
                n281 = Array Subset(array=w490, length=w489) -> (w488:T4[])  [unwired: 1 in]
                n282 = Select(t=w495, s=w494, f=w496) -> (s? t:f=w497:u32)
                n283 = Build Array(w497) -> (w487:u32[])
                n284 = property on="Waveforms" class="Arr (strict)"(error in=w492, "Value"=w488, "Index Values"=w487) -> (error out=w491:errorcluster)  [unwired: 1 in, 1 out]
              }
              frame True {
              }
            }
            n285 = property on="Waveform Graph" class="WFGraph (strict)"(error in=w479) -> (error out=w485:errorcluster, "Value"=w486:sgl[][])  [unwired: 1 in, 1 out]
            n286 = property on="Waveform Graph" class="WFGraph (strict)"(error in=w485, "Val(Sgnl)"=w486) -> (error out=w484:errorcluster)  [unwired: 1 in, 1 out]
          }
          event "Reset Visible Time": Value Change {
            n287 = event-data() -> ()  [unwired: 1 in, 6 out]
            n288 = property on="Max Time" class="DigNum (strict)"(error in=w502) -> (error out=w501:errorcluster, "Value"=w499:dbl)  [unwired: 1 in, 1 out]
            n289 = property on="Time Visible" class="DigNum (strict)"(error in=w501, "Val(Sgnl)"=w499) -> (error out=w500:errorcluster)  [unwired: 1 in, 1 out]
          }
          event "Time Visible": Value Change {
            n290 = event-data() -> ()  [unwired: 1 in, 6 out]
            n291 = property on="Waveform Graph" class="WFGraph (strict)"(error in=w507) -> (error out=w506:errorcluster, "XScale.Minimum"=w505:dbl)  [unwired: 1 in, 1 out]
            n292 = local read "Max Time"() -> (w509:dbl)
            n293 = Add(x=w505, y="Time Visible") -> (x+y=w508:dbl)
            n294 = Less Or Equal?(x=w508, y=w509) -> (x <= y?=w510:bool)
            n295 = case shown="False" w510 {
              tunnel: w509 -> [w511 _]
              tunnel: "Time Visible" -> [w516 _]
              tunnel: w508 -> [_ w519]
              tunnel: w506 -> [w513 w518]
              tunnel: [w515 w517] -> w503
              frame False {
                n296 = property on="Waveform Graph" class="WFGraph (strict)"(error in=w513, "XScale.Maximum"=w511) -> (error out=w512:errorcluster)  [unwired: 1 in, 1 out]
                n297 = Subtract(x=w511, y=w516) -> (x-y=w514:dbl)
                n298 = property on="Waveform Graph" class="WFGraph (strict)"(error in=w512, "XScale.Minimum"=w514) -> (error out=w515:errorcluster)  [unwired: 1 in, 1 out]
              }
              frame True {
                n299 = property on="Waveform Graph" class="WFGraph (strict)"(error in=w518, "XScale.Maximum"=w519) -> (error out=w517:errorcluster)  [unwired: 1 in, 1 out]
              }
            }
          }
        }
      }
    }
    frame Error {
    }
  }
  "error out" <- w18
